vi "queue_selector.vi"(6 "station":T4, 11 "all_config_info_in":T1) -> (3 "queue_out":refnum<queue>)   [LabVIEW 2020]
uses:
  station.ctl
  ini/typedef/PROXY_all_config_info.ctl
  ini/typedef/PROXY_main_ini_file.ctl
  queues/typedef/PROXY_queue_refnums.ctl
  queues/typedef/STATION_queue_element.ctl
  ST_SQL_sequence_state.ctl
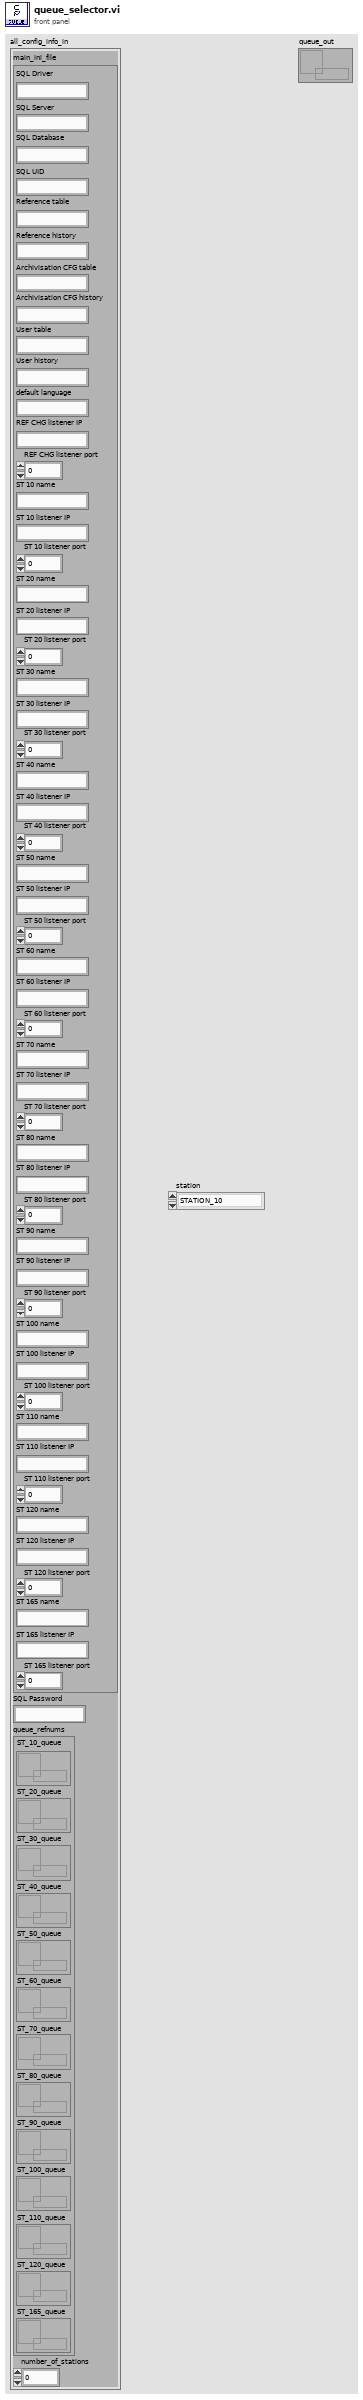
[diagram p1: front panel]
types:
  T1 = typedef "PROXY_all_config_info.ctl" = cluster{"main_ini_file":T2, "SQL Password":string, "queue_refnums":T3, "number_of_stations":i32}
  T2 = typedef "PROXY_main_ini_file.ctl" = cluster{"SQL Driver":string, "SQL Server":string, "SQL Database":string, "SQL UID":string, "Reference table":string, "Reference history":string, "Archivisation CFG table":string, "Archivisation CFG history":string, "User table":string, "User history":string, "default language":string, "REF CHG listener IP":string, "REF CHG listener port":u16, "ST 10 name":string, "ST 10 listener IP":string, "ST 10 listener port":u16, "ST 20 name":string, "ST 20 listener IP":string, "ST 20 listener port":u16, "ST 30 name":string, "ST 30 listener IP":string, "ST 30 listener port":u16, "ST 40 name":string, "ST 40 listener IP":string, "ST 40 listener port":u16, "ST 50 name":string, "ST 50 listener IP":string, "ST 50 listener port":u16, "ST 60 name":string, "ST 60 listener IP":string, "ST 60 listener port":u16, "ST 70 name":string, "ST 70 listener IP":string, "ST 70 listener port":u16, "ST 80 name":string, "ST 80 listener IP":string, "ST 80 listener port":u16, "ST 90 name":string, "ST 90 listener IP":string, "ST 90 listener port":u16, "ST 100 name":string, "ST 100 listener IP":string, "ST 100 listener port":u16, "ST 110 name":string, "ST 110 listener IP":string, "ST 110 listener port":u16, "ST 120 name":string, "ST 120 listener IP":string, "ST 120 listener port":u16, "ST 165 name":string, "ST 165 listener IP":string, "ST 165 listener port":u16}
  T3 = typedef "PROXY_queue_refnums.ctl" = cluster{"ST_10_queue":refnum<queue>, "ST_20_queue":refnum<queue>, "ST_30_queue":refnum<queue>, "ST_40_queue":refnum<queue>, "ST_50_queue":refnum<queue>, "ST_60_queue":refnum<queue>, "ST_70_queue":refnum<queue>, "ST_80_queue":refnum<queue>, "ST_90_queue":refnum<queue>, "ST_100_queue":refnum<queue>, "ST_110_queue":refnum<queue>, "ST_120_queue":refnum<queue>, "ST_165_queue":refnum<queue>}
  T4 = typedef "station.ctl" = enum16{"STATION_10", "STATION_20", "STATION_30", "STATION_40", "STATION_50", "STATION_60", "STATION_70", "STATION_80", "STATION_90", "STATION_100", "STATION_110", "STATION_120", "STATION_165", "MAIN"}
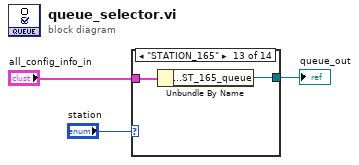
[diagram p0: block diagram]
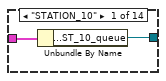
[diagram p2: hidden frame]
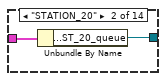
[diagram p3: hidden frame]
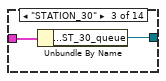
[diagram p4: hidden frame]
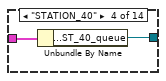
[diagram p5: hidden frame]
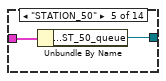
[diagram p6: hidden frame]
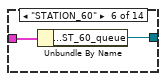
[diagram p7: hidden frame]
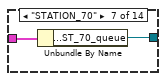
[diagram p8: hidden frame]
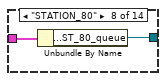
[diagram p9: hidden frame]
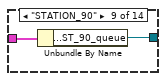
[diagram p10: hidden frame]
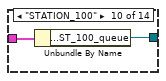
[diagram p11: hidden frame]
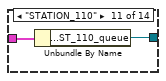
[diagram p12: hidden frame]
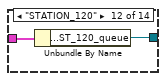
[diagram p13: hidden frame]
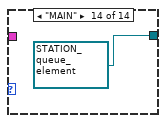
[diagram p14: hidden frame]
diagram:
  n1 = case shown="\"STATION_165\"" "station" {
    tunnel: "all_config_info_in" -> [w5 w7 w9 w11 w13 w15 w17 w19 w21 w23 w25 w27 w29 _]
    tunnel: [w4 w6 w8 w10 w12 w14 w16 w18 w20 w22 w24 w26 w28 refnum<queue> refnum ("ST_30_queue")] -> w1
    frame "STATION_10" {
      n2 = Unbundle By Name(w5) -> ("queue_refnums.ST_10_queue"=w4:refnum<queue>)
    }
    frame "STATION_20" {
      n3 = Unbundle By Name(w7) -> ("queue_refnums.ST_20_queue"=w6:refnum<queue>)
    }
    frame "STATION_30" {
      n4 = Unbundle By Name(w9) -> ("queue_refnums.ST_30_queue"=w8:refnum<queue>)
    }
    frame "STATION_40" {
      n5 = Unbundle By Name(w11) -> ("queue_refnums.ST_40_queue"=w10:refnum<queue>)
    }
    frame "STATION_50" {
      n6 = Unbundle By Name(w13) -> ("queue_refnums.ST_50_queue"=w12:refnum<queue>)
    }
    frame "STATION_60" {
      n7 = Unbundle By Name(w15) -> ("queue_refnums.ST_60_queue"=w14:refnum<queue>)
    }
    frame "STATION_70" {
      n8 = Unbundle By Name(w17) -> ("queue_refnums.ST_70_queue"=w16:refnum<queue>)
    }
    frame "STATION_80" {
      n9 = Unbundle By Name(w19) -> ("queue_refnums.ST_80_queue"=w18:refnum<queue>)
    }
    frame "STATION_90" {
      n10 = Unbundle By Name(w21) -> ("queue_refnums.ST_90_queue"=w20:refnum<queue>)
    }
    frame "STATION_100" {
      n11 = Unbundle By Name(w23) -> ("queue_refnums.ST_100_queue"=w22:refnum<queue>)
    }
    frame "STATION_110" {
      n12 = Unbundle By Name(w25) -> ("queue_refnums.ST_110_queue"=w24:refnum<queue>)
    }
    frame "STATION_120" {
      n13 = Unbundle By Name(w27) -> ("queue_refnums.ST_120_queue"=w26:refnum<queue>)
    }
    frame "STATION_165" {
      n14 = Unbundle By Name(w29) -> ("queue_refnums.ST_165_queue"=w28:refnum<queue>)
    }
    frame "MAIN" {
    }
  }
  "queue_out" <- w1
